vi "Script Add Constant VI --Class.vi"(4 "Project Ref":refnum<vi>, 6 "App Ref":refnum<vi>, 7 "Constant VI Name":string="TESTING.vi", 8 "error in":errorcluster, 9 "Constant VI Args":refnum<vi>, 10 "Class Reference":refnum<vi>) -> (0 "error out":errorcluster, 3 "Constant VI Path":path)   [LabVIEW 2020, in "ConstantErrorsMaker.lvlib"]
uses:
  ConstantErrorsMaker.lvlib
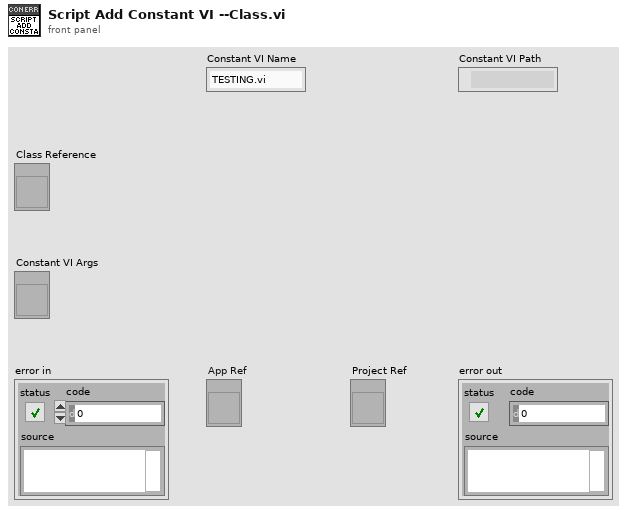
[diagram p1: front panel]
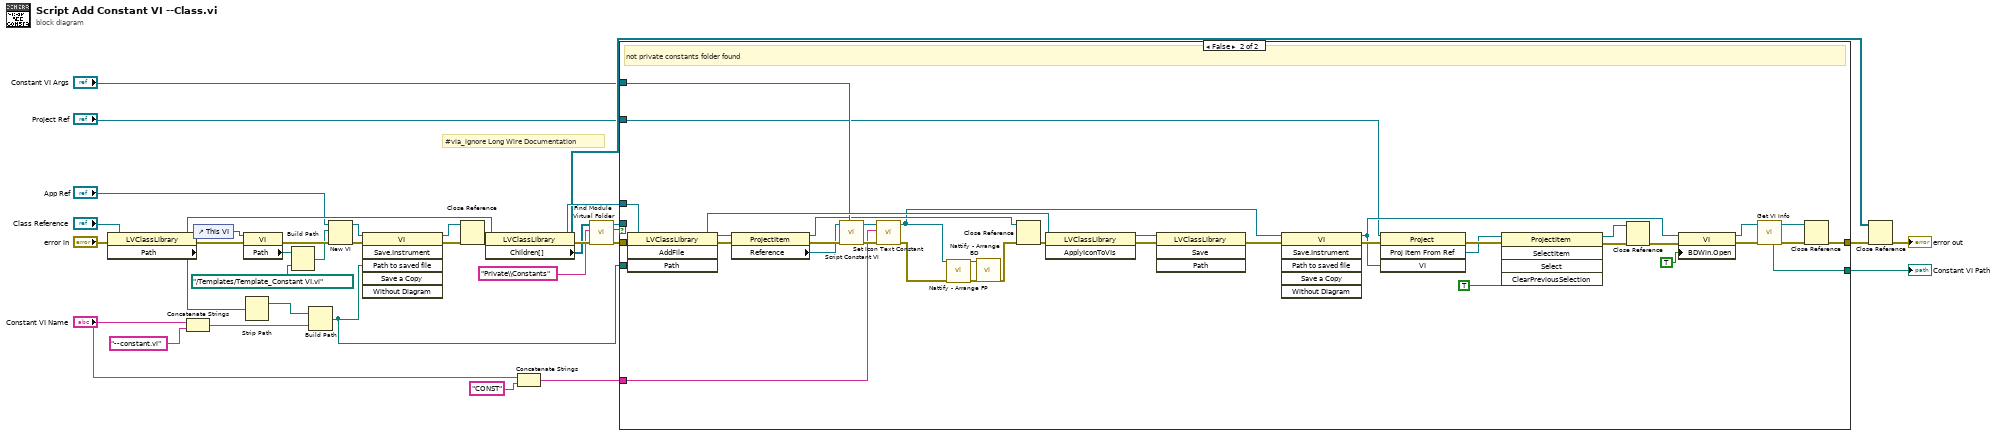
[diagram p0: block diagram]
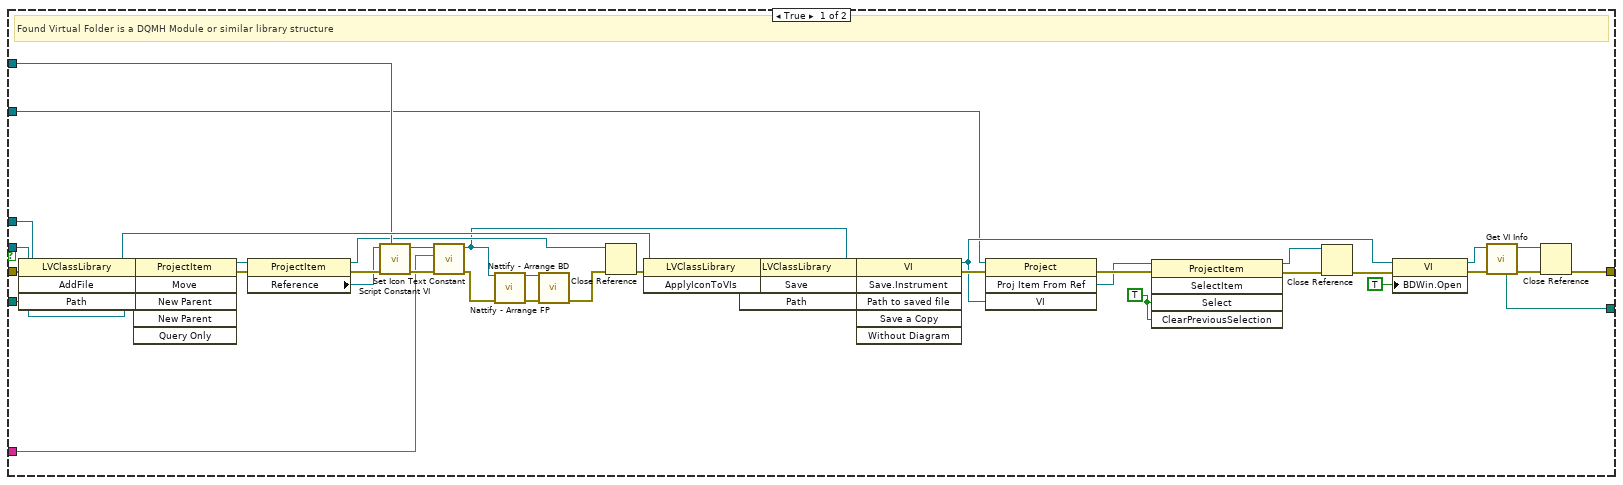
[diagram p2: hidden frame]
diagram:
  # "#via_ignore Long Wire Documentation"
  n1 = property class="LVClassLibrary"(reference="Class Reference", error in="error in") -> (reference out=w24:refnum<vi>, error out=w32:errorcluster, "Path"=w13:path)
  n2 = Concatenate Strings("Constant VI Name", "--constant.vi" ("input 1")) -> (w12:string)
  n3 = control-ref of="This VI"() -> (w11:refnum<vi>)
  n4 = property class="VI"(reference=w11, error in=w32) -> (error out=w26:errorcluster, "Path"=w10:path)  [unwired: 1 out]
  n5 = Strip Path(path=w13) -> (stripped path=w15:path)  [unwired: 1 out]
  n6 = Build Path(base path=w10, name or relative path=path "../Templates/Template_Constant VI.vi") -> (appended path=w9:path)
  n7 = Build Path(base path=w15, name or relative path=w12) -> (appended path=w14:path)
  n8 = New VI(8:w26, 10:w9, 11:"App Ref") -> (0:w29:errorcluster, 3:w17:refnum<vi>)  [unwired: 4 in]
  n9 = invoke class="VI" method="Save.Instrument"(reference=w17, error in=w29, "Path to saved file"=w14) -> (reference out=w7:refnum<vi>, error out=w27:errorcluster)  [unwired: 3 in, 4 out]
  n10 = Close Reference(reference=w7, error in (no error)=w27) -> (error out=w28:errorcluster)
  n11 = property class="LVClassLibrary"(reference=w24, error in=w28) -> (reference out=w25:refnum<vi>, error out=w34:errorcluster, "Children[]"=w21:refnum<vi>[])
  n12 = Concatenate Strings("Constant VI Name", "CONST" ("string")) -> (w3:string)
  n13 = call "Find Module Virtual Folder.vi"("error in"=w34, "Virtual Folder"="Private\\Constants", "Children"=w21) -> ("error out"=w33:errorcluster, "Found?"=w22:bool, "ProjectItem out"=w23:refnum<vi>)  [unwired: 6 in]
  n14 = case shown="False" w22 {
    tunnel: [w65 w104] -> w35
    tunnel: w25 -> [w58 w97]
    tunnel: w33 -> [w76 w114]
    tunnel: w23 -> [w56 _]
    tunnel: "Constant VI Args" -> [w52 w92]
    tunnel: w14 -> [w53 w93]
    tunnel: w3 -> [w45 w86]
    tunnel: "Project Ref" -> [w40 w82]
    tunnel: [w36 w77] -> w1
    frame True {
      w43 = TRUE ("Select")
      # "Found Virtual Folder is a DQMH Module or similar library structure"
      n15 = invoke class="LVClassLibrary" method="AddFile"(reference=w58, error in=w76, "Path"=w53) -> (reference out=w55:refnum<vi>, error out=w75:errorcluster, "AddFile"=w57:refnum<vi>)  [unwired: 1 in, 1 out]
      n16 = invoke class="ProjectItem" method="Move"(reference=w57, error in=w75, "New Parent"=w56) -> (reference out=w50:refnum<vi>, error out=w72:errorcluster)  [unwired: 3 in, 4 out]
      n17 = property class="ProjectItem"(reference=w50, error in=w72) -> (reference out=w49:refnum<vi>, error out=w60:errorcluster, "Reference"=w39:refnum<vi>)
      n18 = call "Script Constant VI.vi"("Custom Argument Window"=w52, "error in"=w60, "VI Reference"=w39) -> ("error out"=w71:errorcluster, "VI reference"=w51:refnum<vi>)  [unwired: 7 in]
      n19 = call "Set Icon Text Constant.vi"("error in"=w71, "Text"=w45, "VI in"=w51) -> ("error out"=w69:errorcluster, "VI out"=w47:refnum<vi>)  [unwired: 7 in]
      n20 = call "Nattify - Arrange FP.vi"("VI in"=w47, "error in"=w69) -> ("VI out"=w48:refnum<vi>, "error out"=w70:errorcluster)  [unwired: 12 in]
      n21 = call "Nattify - Arrange BD.vi"("VI in"=w48, "error in"=w70) -> ("error out"=w67:errorcluster)  [unwired: 13 in]
      n22 = Close Reference(reference=w49, error in (no error)=w67) -> (error out=w73:errorcluster)
      n23 = invoke class="LVClassLibrary" method="ApplyIconToVIs"(reference=w55, error in=w73) -> (reference out=w54:refnum<vi>, error out=w74:errorcluster)  [unwired: 1 in, 1 out]
      n24 = invoke class="LVClassLibrary" method="Save"(reference=w54, error in=w74) -> (error out=w66:errorcluster)  [unwired: 2 in, 3 out]
      n25 = invoke class="VI" method="Save.Instrument"(reference=w47, error in=w66) -> (reference out=w42:refnum<vi>, error out=w63:errorcluster)  [unwired: 4 in, 4 out]
      n26 = invoke class="Project" method="Proj Item From Ref"(reference=w40, error in=w63, "VI"=w42) -> (error out=w64:errorcluster, "ProjItemFromRef"=w44:refnum<vi>)  [unwired: 1 in, 2 out]
      n27 = invoke class="ProjectItem" method="SelectItem"(reference=w44, error in=w64, "Select"=w43, "ClearPreviousSelection"=w43) -> (reference out=w41:refnum<vi>, error out=w62:errorcluster)  [unwired: 1 in, 3 out]
      n28 = Close Reference(reference=w41, error in (no error)=w62) -> (error out=w61:errorcluster)
      n29 = property class="VI"(reference=w42, error in=w61, "BDWin.Open"=TRUE ("Block Diagram Window:Open")) -> (reference out=w38:refnum<vi>, error out=w68:errorcluster)
      n30 = call "Get VI Info.vi"("error in"=w68, "VI in"=w38) -> ("error out"=w59:errorcluster, "VI out"=w37:refnum<vi>, "VI Path"=w36:path)  [unwired: 4 in, 3 out]
      n31 = Close Reference(reference=w37, error in (no error)=w59) -> (error out=w65:errorcluster)
    }
    frame False {
      w84 = TRUE ("Select")
      # "not private constants folder found"
      n32 = invoke class="LVClassLibrary" method="AddFile"(reference=w97, error in=w114, "Path"=w93) -> (reference out=w95:refnum<vi>, error out=w103:errorcluster, "AddFile"=w96:refnum<vi>)  [unwired: 1 in, 1 out]
      n33 = property class="ProjectItem"(reference=w96, error in=w103) -> (reference out=w90:refnum<vi>, error out=w110:errorcluster, "Reference"=w80:refnum<vi>)
      n34 = call "Script Constant VI.vi"("Custom Argument Window"=w92, "error in"=w110, "VI Reference"=w80) -> ("error out"=w111:errorcluster, "VI reference"=w91:refnum<vi>)  [unwired: 7 in]
      n35 = call "Set Icon Text Constant.vi"("error in"=w111, "Text"=w86, "VI in"=w91) -> ("error out"=w108:errorcluster, "VI out"=w88:refnum<vi>)  [unwired: 7 in]
      n36 = call "Nattify - Arrange FP.vi"("VI in"=w88, "error in"=w108) -> ("VI out"=w89:refnum<vi>, "error out"=w109:errorcluster)  [unwired: 12 in]
      n37 = call "Nattify - Arrange BD.vi"("VI in"=w89, "error in"=w109) -> ("error out"=w106:errorcluster)  [unwired: 13 in]
      n38 = Close Reference(reference=w90, error in (no error)=w106) -> (error out=w112:errorcluster)
      n39 = invoke class="LVClassLibrary" method="ApplyIconToVIs"(reference=w95, error in=w112) -> (reference out=w94:refnum<vi>, error out=w113:errorcluster)  [unwired: 1 in, 1 out]
      n40 = invoke class="LVClassLibrary" method="Save"(reference=w94, error in=w113) -> (error out=w105:errorcluster)  [unwired: 2 in, 3 out]
      n41 = invoke class="VI" method="Save.Instrument"(reference=w88, error in=w105) -> (reference out=w83:refnum<vi>, error out=w101:errorcluster)  [unwired: 4 in, 4 out]
      n42 = invoke class="Project" method="Proj Item From Ref"(reference=w82, error in=w101, "VI"=w83) -> (error out=w102:errorcluster, "ProjItemFromRef"=w85:refnum<vi>)  [unwired: 1 in, 2 out]
      n43 = invoke class="ProjectItem" method="SelectItem"(reference=w85, error in=w102, "Select"=w84, "ClearPreviousSelection"=w84) -> (reference out=w81:refnum<vi>, error out=w100:errorcluster)  [unwired: 1 in, 3 out]
      n44 = Close Reference(reference=w81, error in (no error)=w100) -> (error out=w99:errorcluster)
      n45 = property class="VI"(reference=w83, error in=w99, "BDWin.Open"=TRUE ("Block Diagram Window:Open")) -> (reference out=w79:refnum<vi>, error out=w107:errorcluster)
      n46 = call "Get VI Info.vi"("error in"=w107, "VI in"=w79) -> ("error out"=w98:errorcluster, "VI out"=w78:refnum<vi>, "VI Path"=w77:path)  [unwired: 4 in, 3 out]
      n47 = Close Reference(reference=w78, error in (no error)=w98) -> (error out=w104:errorcluster)
    }
  }
  "Constant VI Path" <- w1
  n48 = Close Reference(reference=w21, error in (no error)=w35) -> (error out=→"error out":errorcluster)
